vi "ActDriveStraight.vi"(9 "FirstTime":bool, 10 "MaxSpeed (ft/s)":dbl, 11 "Dist (ft)":dbl) -> (1 "XSpeedDemand":dbl, 3 "Done":bool)   [LabVIEW 2020]
doc: "Robot will drive forward straight a set distance utilizing position control \n\nInputs:\n-- MaxSpeed -- Double -- in ft/s, the MaxSpeed the robot can go -- \n-- Dist (ft) -- Double -- Distance in feet you want the robot to go -- \n-- FirstTime -- Boolean -- Input true the first time this function is called, sets the target position -- \n\nOutputs:\n-- Done -- Bool -- has the robot reached its target distance\n-- LeftSpeedDemand -- Double -- Speed Demand for left drive train inorder to reach target -- \n-- RightSpeedDemand -- Double -- Speed Demand for left drive train inorder to reach target --"
uses:
  <vilib>/Rock Robotics/Network Tables/NT Write Number.vi
  <vilib>/Rock Robotics/WPI/ThirdParty/JAS_Junk/TrajLib/Trajectory_Library.lvlib
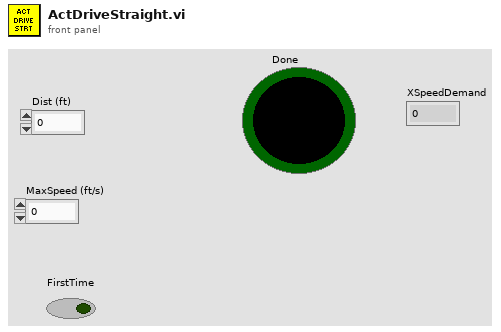
[diagram p1: front panel]
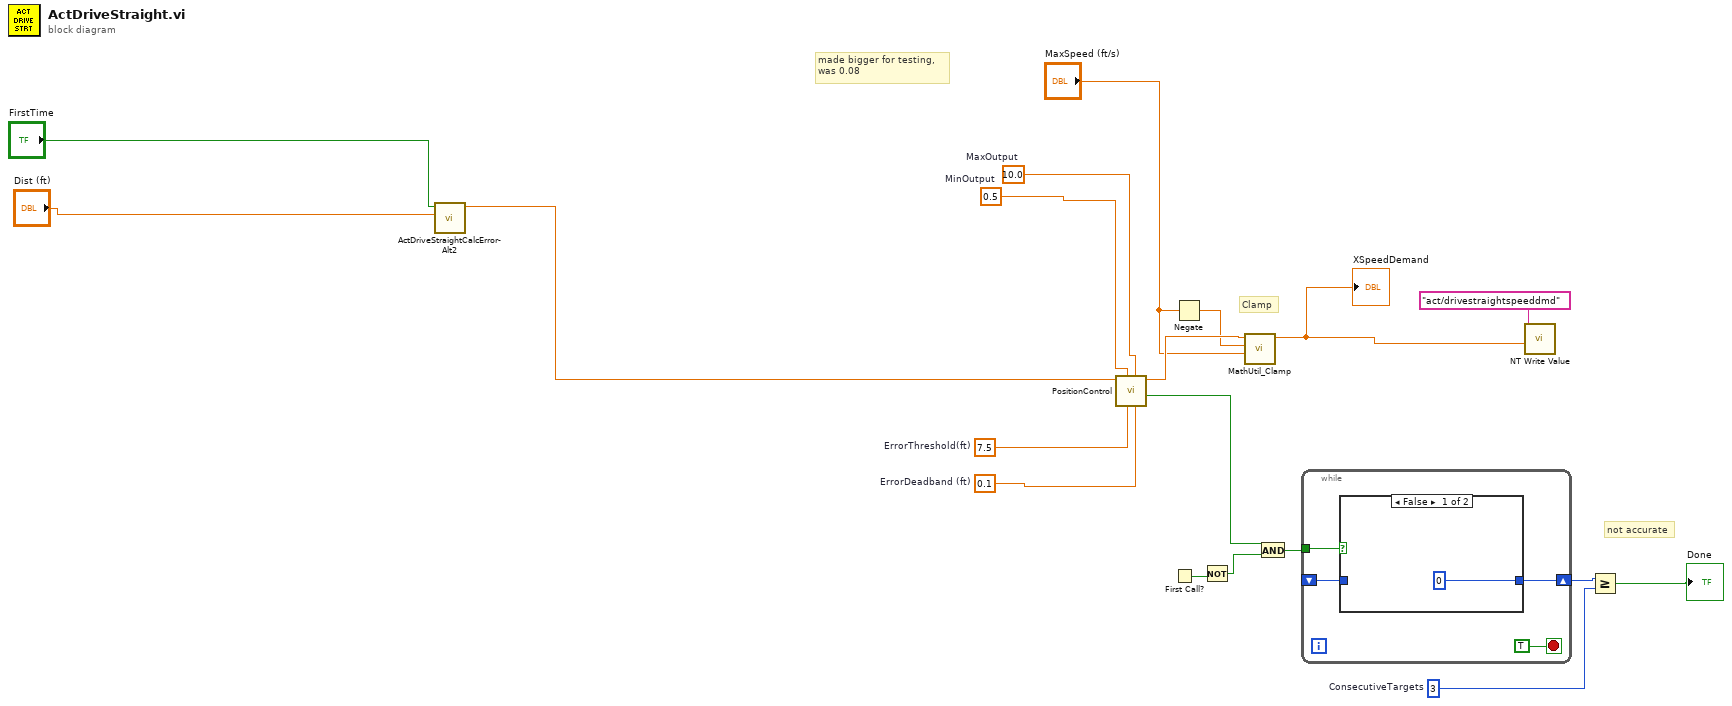
[diagram p0: block diagram]
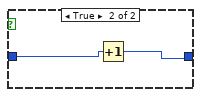
[diagram p2: hidden frame]
diagram:
  w13 = 3  # ConsecutiveTargets
  w8 = 10.0  # MaxOutput
  w7 = 0.5  # MinOutput
  w5 = 0.1  # ErrorDeadband (ft)
  w6 = 7.5  # ErrorThreshold(ft)
  # "not accurate"
  # "made bigger for testing, \nwas 0.08"
  # "Clamp"
  n1 = call "ActDriveStraightCalcError-Alt2.vi"("Dist (ft)"="Dist (ft)", "FirstTime"="FirstTime") -> ("Numeric"=w1:dbl)  [unwired: 9 in]
  n2 = call "PositionControl.vi"("deadband"=w5, "maxdemand"=w8, "threshold"=w6, "mindemand"=w7, "Error"=w1) -> ("on target"=w4:bool, "output variable"=w19:dbl)  [unwired: 5 in]
  n3 = First Call?() -> (First Call?: T/F=w12:bool)
  n4 = Negate(x="MaxSpeed (ft/s)") -> (-x=w18:dbl)
  n5 = Not(x=w12) -> (.not. x?=w10:bool)
  n6 = call <vilib>:"MathUtil_Clamp.vi"("High Limit"="MaxSpeed (ft/s)", "Low Limit"=w18, "Value"=w19) -> ("Result"=w16:dbl)  [unwired: 8 in]
  "XSpeedDemand" <- w16
  n7 = And(x=w4, y=w10) -> (x .and. y?=w11:bool)
  n8 = while {
    tunnel: w11 -> [w22]
    shift-right: [w21] -> w14
    shift-left: _ -> [w20]
    stop <- TRUE stop-if-true
    n9 = case shown="False" w22 {
      tunnel: [0 w25] -> w21
      tunnel: w20 -> [_ w26]
      frame False {
      }
      frame True {
        n10 = Increment(x=w26) -> (x+1=w25:i32)
      }
    }
  }
  n11 = call-poly <vilib>:"NT Write Value.vi"("value"=w16, "name"="act/drivestraightspeeddmd") -> ()  [unwired: 9 in, 1 out]
  n12 = Greater Or Equal?(x=w14, y=w13) -> (x >= y?=→"Done":bool)
